vi "Release.vi"(8 "error in (no error)":errorcluster) -> (0 "error out":errorcluster)   [LabVIEW 2016, in "Log4Lv.lvlib"]
doc: "Use this template to build a VI to use as a subVI."
uses:
  Log4Lv.lvlib
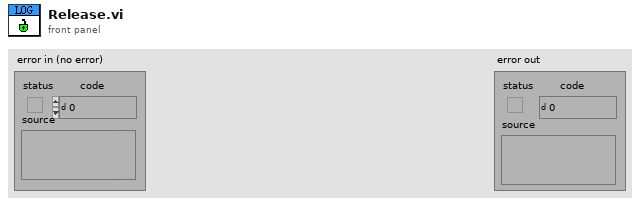
[diagram p1: front panel]
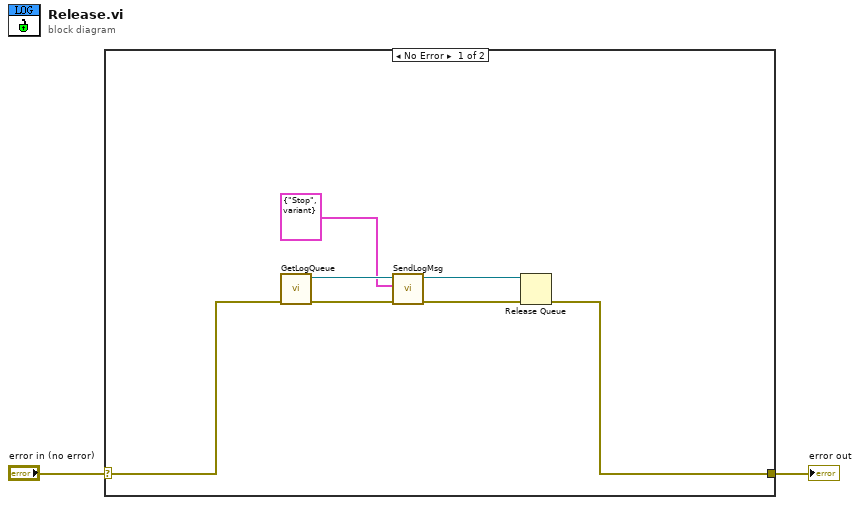
[diagram p0: block diagram]
diagram:
  n1 = case shown="No Error" "error in (no error)" {
    selector: "error in (no error)" -> [w7 w10]
    tunnel: [w4 w10] -> w1
    frame No Error {
      n2 = call "GetLogQueue.vi"("error in (no error)"=w7) -> ("error out"=w9:errorcluster, "Queue Out"=w8:refnum<queue>)  [unwired: 9 in]
      n3 = call "SendLogMsg.vi"("error in (no error)"=w9, "LogMsg"=cluster{"Cmd":string, "Data":variant} {"Cmd"="Stop", "Data"=variant}, "Queue In"=w8) -> ("error out"=w5:errorcluster, "Queue Out"=w3:refnum<queue>)  [unwired: 7 in]
      n4 = Release Queue(queue=w3, error in (no error)=w5) -> (error out=w4:errorcluster)  [unwired: 1 in, 2 out]
    }
    frame Error {
    }
  }
  "error out" <- w1
